vi "Arithmetic Operation.vi"(9 "z":dbl, 10 "y":dbl, 11 "x":dbl) -> (3 "(x+y)*z":dbl)   [LabVIEW 2023]
doc: "Demonstrates the different cases when the number of input value permutations is larger than, equal to, or smaller than the size of vectors assigned to expected values in an arithmetic operation instance."
panel:
  # "Overview: Demonstrates the different cases when the number of input value permutations is larger than, equal to, or smaller than the size of vectors assigned to expected values in an arithmetic operation instance.\nRequirements: LabVIEW Full Development System, Unit Test Framework Toolkit\nInstructions:\n1.  Execute all the four test files for the Arithmetic Operation VI in this project, which are Arithmetic Operation_Error.lvtest, Arithmetic Operation_Fail.lvtest, Arithmetic Operation_Pass.lvtest, Arithmetic Operation_Warn.lvtest. In the Project Explorer window, right-click Arithmetic Operation.vi to select Unit Tests>>Run from the shortcut menu.\n2.  View the test results in the Unit Test Framework Results window, which shows that two tests passed, one test failed, and one test reported error during test execution.\n3.  In the Project Explorer window, double-click each of the four test files to display the Test Cases page of the Test Properties dialog box. You can see that test vectors x, y, and z in Arithmetic Operation.lvvect > are respectively assigned to the x, y, and z controls of this VI with no index.\n4.  In the Test Properties window, select Test Vectors from the Category list to display the values of each test vector.\n5.  Return to this VI. Display the block diagram by selecting Windows>>Show Block Diagram. Read the comments on the block diagram to understand how LabVIEW generates permutations for input values when test vectors are assigned to the inputs of the VI under test.\n6.  Return to the Test Properties dialog box and read the comments on the Test Cases page to understand why a test passes, fails, reports an error, or displays a warning icon."
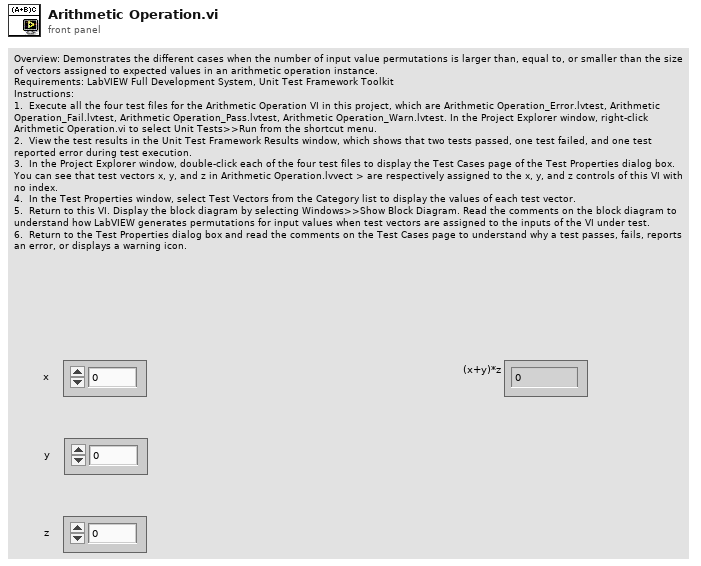
[diagram p1: front panel]
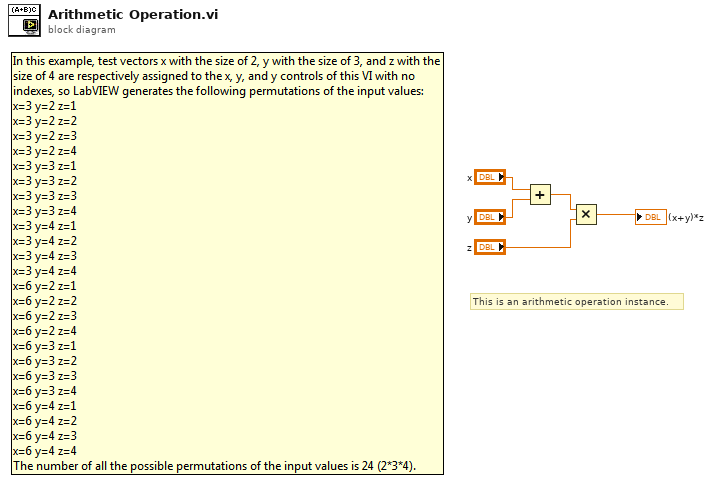
[diagram p0: block diagram]
diagram:
  # "This is an arithmetic operation instance."
  n1 = Add(x="x", y="y") -> (x+y=w3:dbl)
  n2 = Multiply(x=w3, y="z") -> (x*y=→"(x+y)*z":dbl)
